vi "Close.vi"(8 "error in (no error)":errorcluster, 11 "SPI Ref In":T1={"myRIO Reference"={"myRIO Model"=enum."Unknown", "myRIO Hardware Reference"={"Generic FPGA Reference"=refnum, "Allow multiple opens"=FALSE}}, "SPI Channels Enum"=enum."Not Connected", "SPI Configuration"={"Frequency [Hz]"=0.0, "Clock Phase"=enum."Leading", "Clock Polarity"=enum."Low", "Data Direction"=enum."Most significant bit first", "Frame Length"=8}} {"SPI Configuration"."Frame Length" min=1 max=16}) -> (0 "error out":errorcluster)   [LabVIEW 2021, in "SPI.lvlib"]
doc: "Closes the reference to a serial peripheral interface (SPI) channel. This VI also disables the SPI channel and resets the configuration of the channel."
uses:
  <vilib>/myRIO/Instrument Drivers/Onboard IO/SPI/SPI.lvlib
  <vilib>/myRIO/Instrument Drivers/Onboard IO/SPI/typedefs/SPI Reference.ctl
  <vilib>/myRIO/Common/Instrument Driver Framework/Utilities/typedefs/myRIO Generic Hardware Reference.ctl
  <vilib>/myRIO/Common/Instrument Driver Framework/Utilities/typedefs/Hardware Version Enum.ctl
  <vilib>/myRIO/Common/Instrument Driver Framework/Utilities/typedefs/myRIO v1.0 Reference.ctl
  <vilib>/myRIO/Common/Instrument Driver Framework/Utilities/typedefs/Generic FPGA Reference.ctl
  <vilib>/myRIO/Common/Instrument Driver Framework/myRIO v1.0/SPI/typedefs/SPI Channels Enum.ctl
  <vilib>/myRIO/Instrument Drivers/Onboard IO/SPI/typedefs/SPI Configuration.ctl
  <vilib>/myRIO/Common/Instrument Driver Framework/myRIO v1.0/SPI/typedefs/SPI Clock Phase.ctl
  <vilib>/myRIO/Common/Instrument Driver Framework/myRIO v1.0/SPI/typedefs/SPI Clock Polarity.ctl
  <vilib>/myRIO/Common/Instrument Driver Framework/myRIO v1.0/SPI/typedefs/SPI Data Direction.ctl
  <vilib>/myRIO/Common/Instrument Driver Framework/myRIO v1.0/SPI/typedefs/SPI Frame Length.ctl
  <vilib>/myRIO/Common/Instrument Driver Framework/myRIO v1.0/SPI/vis/myRIO v1.0 Unreserve SPI.vi
  <vilib>/myRIO/Common/Instrument Driver Framework/roboRIO v1.0/SPI/vis/roboRIO v1.0 Unreserve SPI.vi
  <vilib>/myRIO/Common/Instrument Driver Framework/ELVIS III v1.0/SPI/vis/ELVIS III v1.0 Unreserve SPI.vi
  <vilib>/myRIO/Common/Instrument Driver Framework/myRIO v1.0/SPI/vis/myRIO v1.0 Build MUX Configuration SPI.vi
  <vilib>/myRIO/Common/Instrument Driver Framework/myRIO v1.0/Resource Manager/vis/myRIO v1.0 Unreserve Channel List.vi
  <vilib>/myRIO/Common/Instrument Driver Framework/roboRIO v1.0/Resource Manager/vis/roboRIO v1.0 Unreserve Channel List.vi
  <vilib>/myRIO/Common/Instrument Driver Framework/roboRIO v1.0/SPI/vis/roboRIO v1.0 Build MUX Configuration SPI.vi
  <vilib>/myRIO/Common/Instrument Driver Framework/ELVIS III v1.0/SPI/vis/ELVIS III v1.0 Build MUX Configuration SPI.vi
  <vilib>/myRIO/Common/Instrument Driver Framework/myRIO v1.0/Resource Manager/vis/myRIO v1.0 Create Configuration List.vi
  <vilib>/myRIO/Common/Instrument Driver Framework/myRIO v1.0/Resource Manager/vis/myRIO v1.0 Unreserve Channel.vi
  <vilib>/myRIO/Common/Instrument Driver Framework/roboRIO v1.0/Resource Manager/vis/roboRIO v1.0 Unreserve Channel.vi
  <vilib>/myRIO/Common/Instrument Driver Framework/ELVIS III v1.0/Resource Manager/vis/ELVIS III v1.0 Create Configuration List.vi
  <vilib>/myRIO/Common/Instrument Driver Framework/myRIO v1.0/Resource Manager/vis/myRIO v1.0 Build Mutex Name.vi
  <vilib>/myRIO/Common/Instrument Driver Framework/roboRIO v1.0/Resource Manager/vis/roboRIO v1.0 Build Mutex Name.vi
  <vilib>/myRIO/Common/Instrument Driver Framework/myRIO v1.0/SPI/vis/myRIO v1.0 Shutdown SPI.vi
  <vilib>/myRIO/Common/Instrument Driver Framework/myRIO v1.0/Resource Manager/vis/myRIO v1.0 Configure IO.vi
  <vilib>/myRIO/Common/Instrument Driver Framework/Utilities/vis/Configuration Manager.vi
  <vilib>/myRIO/Common/Instrument Driver Framework/Utilities/vis/IO Manager.vi
  <vilib>/myRIO/Common/Instrument Driver Framework/roboRIO v1.0/SPI/vis/roboRIO v1.0 Shutdown SPI.vi
  <vilib>/myRIO/Common/Instrument Driver Framework/roboRIO v1.0/Resource Manager/vis/roboRIO v1.0 Configure IO.vi
  <vilib>/myRIO/Common/Instrument Driver Framework/ELVIS III v1.0/Resource Manager/vis/ELVIS III v1.0 Configure IO.vi
  <vilib>/myRIO/Common/Instrument Driver Framework/ELVIS III v1.0/Resource Manager/vis/ELVIS III v1.0 Unreserve Channel List.vi
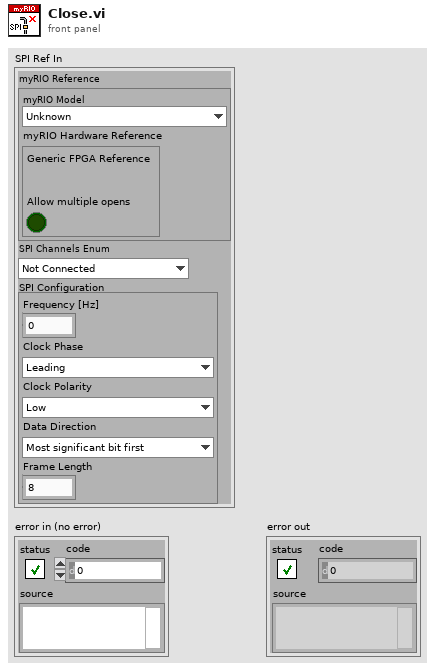
[diagram p1: front panel]
types:
  T1 = typedef "SPI.lvlib/SPI Reference.ctl" = cluster{"myRIO Reference":T2, "SPI Channels Enum":T6, "SPI Configuration":T7}
  T2 = typedef "myRIO Generic Hardware Reference.ctl" = cluster{"myRIO Model":T3, "myRIO Hardware Reference":T4}
  T3 = typedef "Hardware Version Enum.ctl" = enum16{"Unknown", "myRIO-1900", "myRIO-1950", "roboRIO", "NI ELVIS RIO CM", "ELVIS III"}
  T4 = typedef "myRIO v1.0 Reference.ctl" = cluster{"Generic FPGA Reference":T5, "Allow multiple opens":bool}
  T5 = typedef "Generic FPGA Reference.ctl" = refnum<k20>
  T6 = typedef "SPI Channels Enum.ctl" = enum16{"Not Connected", "A/SPI", "B/SPI", "SPI/SPI"}
  T7 = typedef "SPI.lvlib/SPI Configuration.ctl" = cluster{"Frequency [Hz]":dbl, "Clock Phase":T8, "Clock Polarity":T9, "Data Direction":T10, "Frame Length":T11}
  T8 = typedef "SPI Clock Phase.ctl" = enum8{"Leading", "Trailing"}
  T9 = typedef "SPI Clock Polarity.ctl" = enum8{"Low", "High"}
  T10 = typedef "SPI Data Direction.ctl" = enum8{"Most significant bit first", "Least significant bit first"}
  T11 = typedef "SPI Frame Length.ctl" = u8
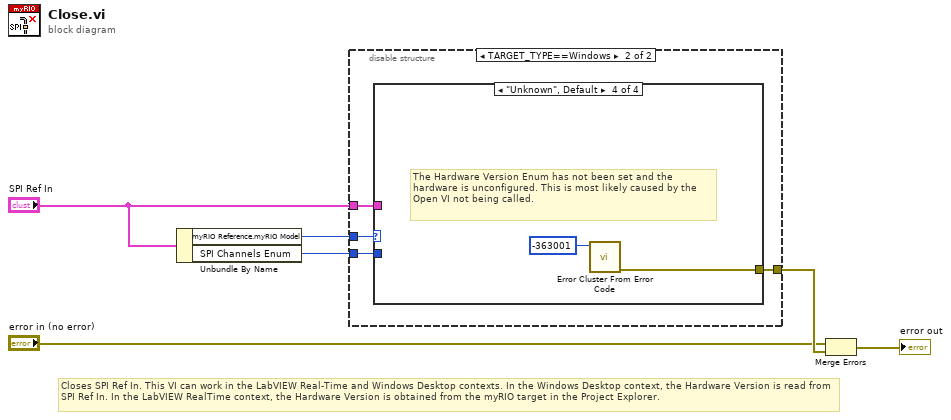
[diagram p0: block diagram]
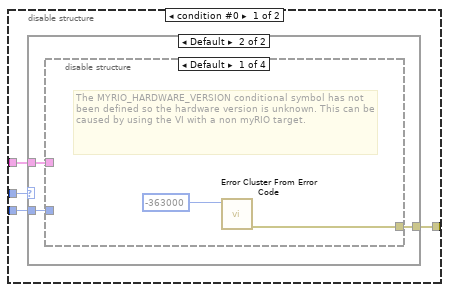
[diagram p2: hidden frame]
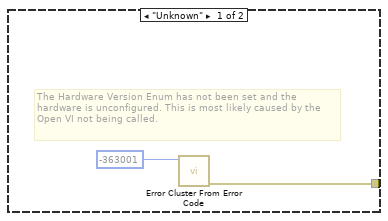
[diagram p3: hidden frame]
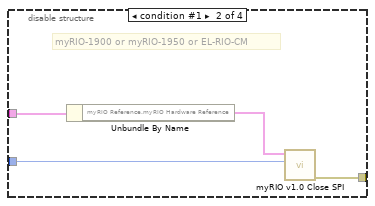
[diagram p4: hidden frame]
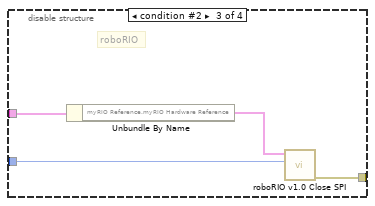
[diagram p5: hidden frame]
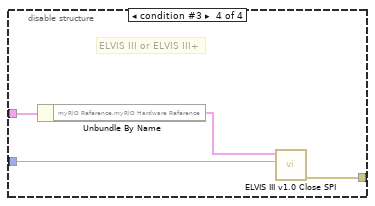
[diagram p6: hidden frame]
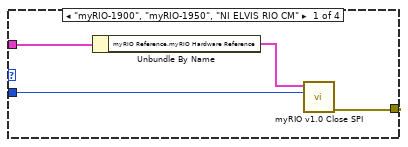
[diagram p7: hidden frame]
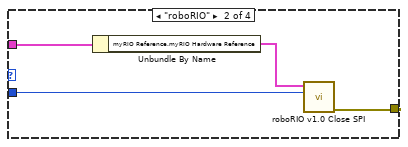
[diagram p8: hidden frame]
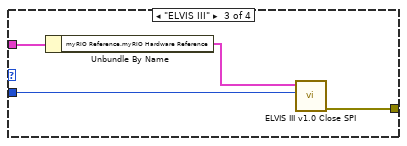
[diagram p9: hidden frame]
diagram:
  # "Closes SPI Ref In. This VI can work in the LabVIEW Real-Time and Windows Desktop contexts. In the Windows Desktop context, the Hardware Version is read from SPI Ref In. In the LabVIEW RealTime context, the Hardware Version is obtained from the myRIO target in the Project Explorer."
  n1 = Unbundle By Name("SPI Ref In") -> ("myRIO Reference.myRIO Model"=w2:T3, "SPI Channels Enum"=w1:T6)
  n2 = disable-structure shown="TARGET_TYPE==Windows" {
    disable-tunnel: "SPI Ref In" -> [w10 w32]
    disable-tunnel: [w9 w33] -> w6
    disable-tunnel: w2 -> [w8 w31]
    disable-tunnel: w1 -> [w7 w30]
    frame condition #0 {
      n3 = case shown="Default" w8 {
        tunnel: w10 -> [_ w15]
        tunnel: [w11 w14] -> w9
        tunnel: w7 -> [_ w13]
        frame "Unknown" {
          # "The Hardware Version Enum has not been set and the hardware is unconfigured. This is most likely caused by the Open VI not being called."
          n4 = call <vilib>:"Error Cluster From Error Code.vi"("error code (0)"=-363001) -> ("error out"=w11:errorcluster)  [unwired: 8 in]
        }
        frame Default {
          n5 = disable-structure shown="Default" {
            disable-tunnel: w15 -> [_ w21 w25 w29]
            disable-tunnel: [w16 w20 w24 w26] -> w14
            disable-tunnel: w13 -> [_ w18 w22 w27]
            frame condition #0 (active) {
              # "The MYRIO_HARDWARE_VERSION conditional symbol has not been defined so the hardware version is unknown. This can be caused by using the VI with a non myRIO target."
              n6 = call <vilib>:"Error Cluster From Error Code.vi"("error code (0)"=-363000) -> ("error out"=w16:errorcluster)  [unwired: 8 in]
            }
            frame condition #1 {
              # "myRIO-1900 or myRIO-1950 or EL-RIO-CM"
              n7 = Unbundle By Name(w21) -> ("myRIO Reference.myRIO Hardware Reference"=w19:T4)
              n8 = call <vilib>:"myRIO v1.0 Close SPI.vi"("SPI Channel"=w18, "myRIO Ref In"=w19) -> ("error out"=w20:errorcluster)  [unwired: 9 in]
            }
            frame condition #2 {
              # "roboRIO"
              n9 = Unbundle By Name(w25) -> ("myRIO Reference.myRIO Hardware Reference"=w23:T4)
              n10 = call <vilib>:"roboRIO v1.0 Close SPI.vi"("SPI Channel"=w22, "myRIO Ref In"=w23) -> ("error out"=w24:errorcluster)  [unwired: 9 in]
            }
            frame condition #3 {
              # "ELVIS III or ELVIS III+"
              n11 = Unbundle By Name(w29) -> ("myRIO Reference.myRIO Hardware Reference"=w28:T4)
              n12 = call <vilib>:"ELVIS III v1.0 Close SPI.vi"("SPI Channel"=w27, "myRIO Ref In"=w28) -> ("error out"=w26:errorcluster)  [unwired: 9 in]
            }
          }
        }
      }
    }
    frame condition #1 (active) {
      n13 = case shown="\"Unknown\", Default" w31 {
        tunnel: w32 -> [w37 w41 w45 _]
        tunnel: [w36 w40 w42 w46] -> w33
        tunnel: w30 -> [w34 w38 w43 _]
        frame "myRIO-1900", "myRIO-1950", "NI ELVIS RIO CM" {
          n14 = Unbundle By Name(w37) -> ("myRIO Reference.myRIO Hardware Reference"=w35:T4)
          n15 = call <vilib>:"myRIO v1.0 Close SPI.vi"("SPI Channel"=w34, "myRIO Ref In"=w35) -> ("error out"=w36:errorcluster)  [unwired: 9 in]
        }
        frame "roboRIO" {
          n16 = Unbundle By Name(w41) -> ("myRIO Reference.myRIO Hardware Reference"=w39:T4)
          n17 = call <vilib>:"roboRIO v1.0 Close SPI.vi"("SPI Channel"=w38, "myRIO Ref In"=w39) -> ("error out"=w40:errorcluster)  [unwired: 9 in]
        }
        frame "ELVIS III" {
          n18 = Unbundle By Name(w45) -> ("myRIO Reference.myRIO Hardware Reference"=w44:T4)
          n19 = call <vilib>:"ELVIS III v1.0 Close SPI.vi"("SPI Channel"=w43, "myRIO Ref In"=w44) -> ("error out"=w42:errorcluster)  [unwired: 9 in]
        }
        frame "Unknown", Default {
          # "The Hardware Version Enum has not been set and the hardware is unconfigured. This is most likely caused by the Open VI not being called."
          n20 = call <vilib>:"Error Cluster From Error Code.vi"("error code (0)"=-363001) -> ("error out"=w46:errorcluster)  [unwired: 8 in]
        }
      }
    }
  }
  n21 = Merge Errors("error in (no error)", w6) -> (→"error out":errorcluster)
